vi "Load State Data.vi"(8 "error in (no error)":errorcluster, 11 "TimingControl in":refnum<class "TimingControl.lvclass">) -> (0 "error out":errorcluster, 3 "TimingControl out":refnum<class "TimingControl.lvclass">)   [LabVIEW 2022 SP3, in "ZKTimingControl.lvlib" / "TimingControl.lvclass"]
doc: "The <b>Load State Data VI</b> is a dynamic dispatch VI that must be overwritten in every QControl Class that uses the State Data. If used it must <b>Call Parent Method</b>. This recursively loads the Data Value Reference to the data space for the QControl Class up the inheritance hierarchy that uses the Data Value Reference.\n<b> </b> <b> </b>\n©2016 Q Software Innovations, LLC (QSI)\nwritten by Quentin Alldredge\nproduced in LabVIEW 2015\n\nsupport@qsoftwareinnovations.com\nwww.qsoftwareinnovations.com\n\nAll rights reserved.\n\nRedistribution and use in source and binary forms, with or without modification, are permitted provided that the following conditions are met:\n\n * Redistributions of source code must retain the above copyright notice, this list of conditions and the following disclaimer.\n * Redistributions in binary form must reproduce the above copyright notice, this list of conditions and the following disclaimer in the documentation and/or other materials provided with the distribution.\n * Neither the name of Q Software Innovations, LLC. nor the names of its contributors may be used to endorse or promote products derived from this software without specific prior written permission.\n\nTHIS SOFTWARE IS PROVIDED BY THE COPYRIGHT HOLDERS AND CONTRIBUTORS \"AS IS\" AND ANY EXPRESS OR IMPLIED WARRANTIES, INCLUDING, BUT NOT LIMITED TO, THE IMPLIED WARRANTIES OF MERCHANTABILITY AND FITNESS FOR A PARTICULAR PURPOSE ARE DISCLAIMED. IN NO EVENT SHALL THE COPYRIGHT OWNER OR CONTRIBUTORS BE LIABLE FOR ANY DIRECT, INDIRECT, INCIDENTAL, SPECIAL, EXEMPLARY, OR CONSEQUENTIAL DAMAGES (INCLUDING, BUT NOT LIMITED TO, PROCUREMENT OF SUBSTITUTE GOODS OR SERVICES; LOSS OF USE, DATA, OR PROFITS; OR BUSINESS INTERRUPTION) HOWEVER CAUSED AND ON ANY THEORY OF LIABILITY, WHETHER IN CONTRACT, STRICT LIABILITY, OR TORT (INCLUDING NEGLIGENCE OR OTHERWISE) ARISING IN ANY WAY OUT OF THE USE OF THIS SOFTWARE, EVEN IF ADVISED OF THE POSSIBILITY OF SUCH DAMAGE."
uses:
  TimingControl.lvclass
  State Data.ctl
  TimingControl.lvclass/TimingControl.ctl
  <vilib>/QSI/QControls/QControl Classes/Boolean/Boolean.lvclass
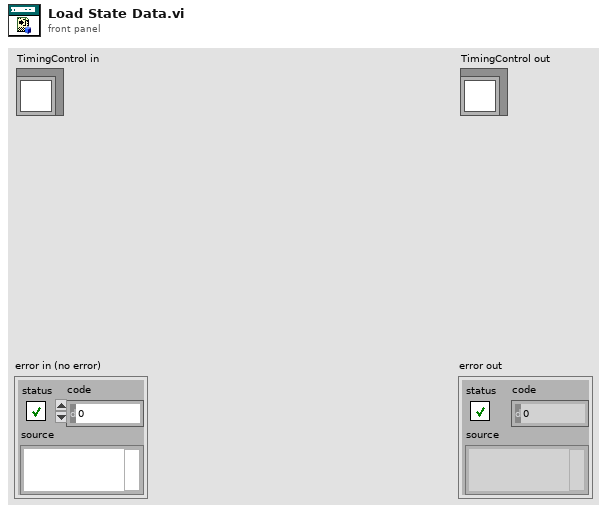
[diagram p1: front panel]
types:
  T1 = typedef "ZKTimingControl.lvlib/TimingControl.lvclass/State Data.ctl" = cluster{"仪器时间":timestamp, "仪器运行状态":bool, "配置文件路径":path, "测量参数":T2, "测试状态":cluster{"启动时间":timestamp, "结束时间":timestamp, "启动次数":dbl}, "配置信息":T3}
  T2 = typedef "ZKTimingControl.lvlib/TimingControl.lvclass/测量参数.ctl" = cluster{"氨氮":bool, "总磷":bool, "总氮":bool, "CODMn":bool, "CODCr":bool, "氟化物":bool, "挥发酚":bool}
  T3 = typedef "ZKTimingControl.lvlib/TimingControl.lvclass/配置信息.ctl" = cluster{"每周启动":T4, "每月启动":T5, "周期模式":T6, "测量参数":T2, "定点周期":T7, "间隔启动":T9, "配置时间":timestamp}
  T4 = typedef "ZKTimingControl.lvlib/TimingControl.lvclass/每周启动.ctl" = enum16{"关闭", "周日", "周一", "周二", "周三", "周四", "周五", "周六"}
  T5 = typedef "ZKTimingControl.lvlib/TimingControl.lvclass/每月启动.ctl" = enum16{"关闭", "1号", "2号", "3号", "4号", "5号", "6号", "7号", "8号", "9号", "10号", "11号", "12号", "13号", "14号", "15号", "16号", "17号", "18号", "19号", "20号", "21号", "22号", "23号", "24号", "25号", "26号", "27号", "28号", "29号", "30号", "31号"}
  T6 = typedef "ZKTimingControl.lvlib/TimingControl.lvclass/周期模式设置.ctl" = enum16{"不启用", "定点模式", "间隔模式"}
  T7 = typedef "ZKTimingControl.lvlib/TimingControl.lvclass/定点周期设置.ctl" = cluster{"启动命令":T8, "启动命令 2":T8, "启动命令 3":T8, "启动命令 4":T8, "启动命令 5":T8, "启动命令 6":T8, "启动命令 7":T8, "启动命令 8":T8, "启动命令 9":T8, "启动命令 10":T8, "启动命令 11":T8, "启动命令 12":T8, "启动命令 13":T8, "启动命令 14":T8, "启动命令 15":T8, "启动命令 16":T8, "启动命令 17":T8, "启动命令 18":T8, "启动命令 19":T8, "启动命令 20":T8, "启动命令 21":T8, "启动命令 22":T8, "启动命令 23":T8, "启动命令 24":T8}
  T8 = typedef "ZKTimingControl.lvlib/TimingControl.lvclass/启动命令选择.ctl" = enum16{"", "加标回收（启动采配水）", "加标回收（不启动采配水）", "水样测试（启动采配水）", "水样测试（不启动采配水）", "平行样测试（启动采配水）", "平行样测试（不启动采配水）", "集成干预测试"}
  T9 = typedef "ZKTimingControl.lvlib/TimingControl.lvclass/间隔启动设置.ctl" = cluster{"启动命令":T8, "启动间隔":dbl, "启动次数":i32}
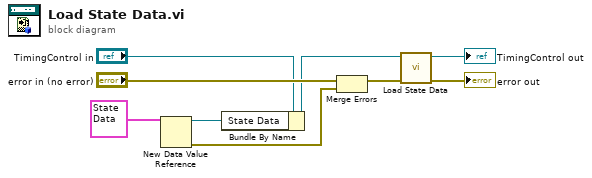
[diagram p0: block diagram]
diagram:
  n1 = New Data Value Reference(data value=T1 {"仪器时间"=timestamp(0 s since 1904-01-01), "仪器运行状态"=FALSE, "配置文件路径"=path "", "测量参数"={"氨氮"=FALSE, "总磷"=FALSE, "总氮"=FALSE, "CODMn"=FALSE, "CODCr"=FALSE, "氟化物"=FALSE, "挥发酚"=FALSE}, "测试状态"={"启动时间"=timestamp(0 s since 1904-01-01), "结束时间"=timestamp(0 s since 1904-01-01), "启动次数"=0.0}, "配置信息"={"每周启动"=enum."关闭", "每月启动"=enum."关闭", "周期模式"=enum."不启用", "测量参数"={"氨氮"=FALSE, "总磷"=FALSE, "总氮"=FALSE, "CODMn"=FALSE, "CODCr"=FALSE, "氟化物"=FALSE, "挥发酚"=FALSE}, "定点周期"={"启动命令"=enum."", "启动命令 2"=enum."", "启动命令 3"=enum."", "启动命令 4"=enum."", "启动命令 5"=enum."", "启动命令 6"=enum."", "启动命令 7"=enum."", "启动命令 8"=enum."", "启动命令 9"=enum."", "启动命令 10"=enum."", "启动命令 11"=enum."", "启动命令 12"=enum."", "启动命令 13"=enum."", "启动命令 14"=enum."", "启动命令 15"=enum."", "启动命令 16"=enum."", "启动命令 17"=enum."", "启动命令 18"=enum."", "启动命令 19"=enum."", "启动命令 20"=enum."", "启动命令 21"=enum."", "启动命令 22"=enum."", "启动命令 23"=enum."", "启动命令 24"=enum.""}, "间隔启动"={"启动命令"=enum."", "启动间隔"=0.0, "启动次数"=0}, "配置时间"=timestamp(0 s since 1904-01-01)}} ("State Data")) -> (data value reference=w4:refnum<data-value>, error out=w2:errorcluster)  [unwired: 1 in]
  n2 = Bundle By Name(cluster="TimingControl in", "State Data"=w4) -> (w5:refnum<class "TimingControl.lvclass">)
  n3 = Merge Errors("error in (no error)", w2) -> (w3:errorcluster)
  n4 = call-parent "Load State Data.vi"("error in (no error)"=w3, "Control in"=w5) -> ("error out"=→"error out":errorcluster, "Control out"=→"TimingControl out":refnum<class "TimingControl.lvclass">)  [unwired: 8 in]
